vi "Set Port HW Entry.vi"(6 "InstrumentHandle_port":u32, 8 "boardresource":T1, 9 "portId":u32, 10 "boardId":u32, 11 "hw_data in":T2) -> (2 "duplicated":bool, 3 "hw_data out":T2)   [LabVIEW 2020, in "AIM664LV.lvlib"]
uses:
  AIM664LV.lvlib
  _controls/hwEntry_data.ctl
  _controls/hwEntryBoardHandleMap.ctl
  _controls/hwEntryBoardResource.ctl
  _controls/hwEntryPortResource.ctl
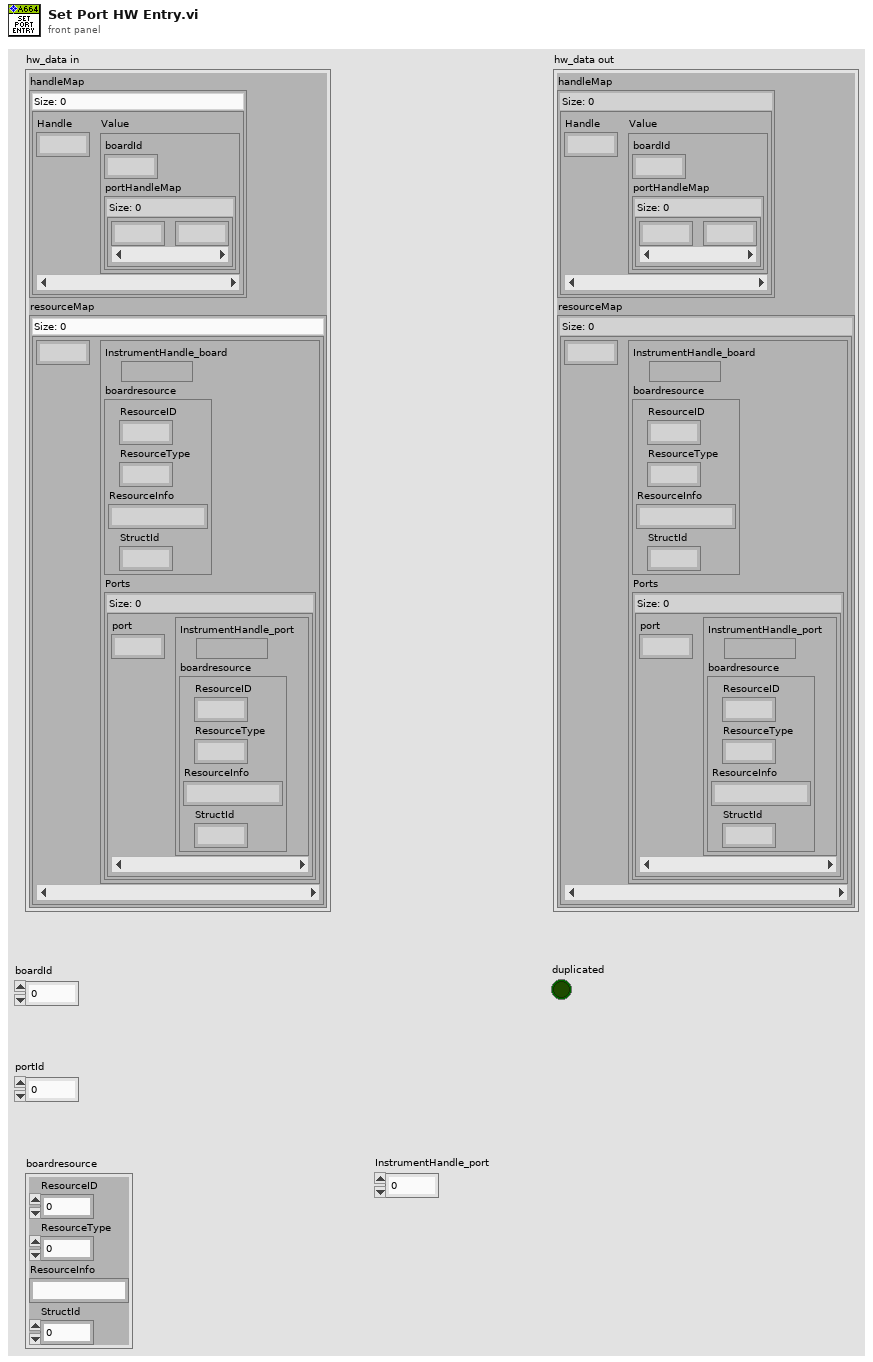
[diagram p1: front panel]
types:
  T1 = cluster{"ResourceID":u32, "ResourceType":u32, "ResourceInfo":string, "StructId":u32}
  T2 = typedef "AIM664LV.lvlib/hwEntry_data.ctl" = cluster{"handleMap":map{u32, T3}, "resourceMap":map{u32, T4}}
  T3 = typedef "AIM664LV.lvlib/hwEntryBoardHandleMap.ctl" = cluster{"boardId":u32, "portHandleMap":map{u32, u32}}
  T4 = typedef "AIM664LV.lvlib/hwEntryBoardResource.ctl" = cluster{"InstrumentHandle_board":u32, "boardresource":cluster{"ResourceID":u32, "ResourceType":u32, "ResourceInfo":string, "StructId":u32}, "Ports":map{u32, T5}}
  T5 = typedef "AIM664LV.lvlib/hwEntryPortResource.ctl" = cluster{"InstrumentHandle_port":u32, "boardresource":cluster{"ResourceID":u32, "ResourceType":u32, "ResourceInfo":string, "StructId":u32}}
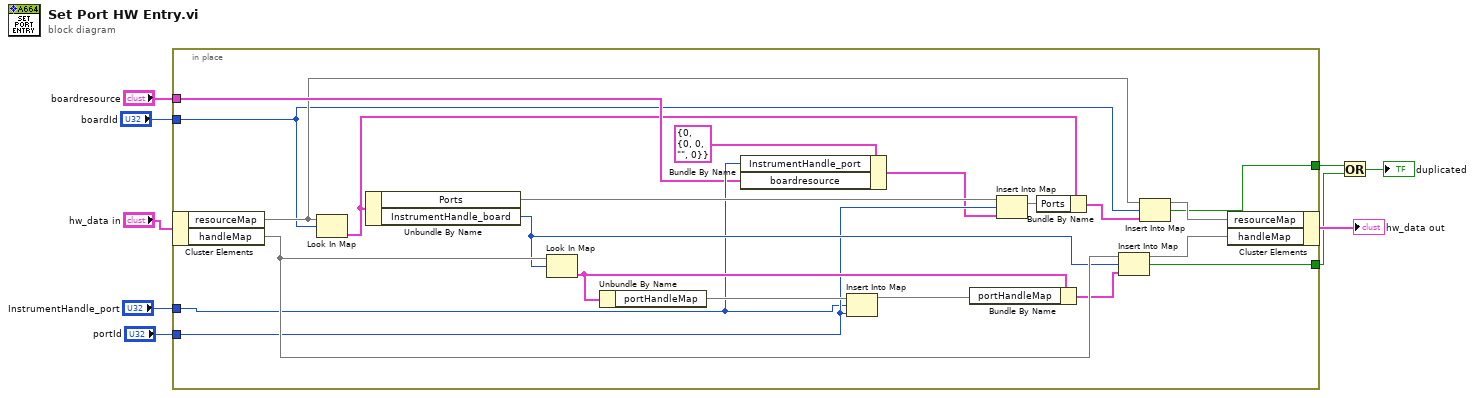
[diagram p0: block diagram]
diagram:
  n1 = in-place {
    in-place-border: "boardId" -> [w13]
    in-place-border: "InstrumentHandle_port" -> [w19]
    in-place-border: "boardresource" -> [w18]
    in-place-border: "portId" -> [w22]
    in-place-border: [w11] -> w2
    in-place-border: [w10] -> w1
    n2 = in-place-cluster #1("hw_data in") -> ("resourceMap"=w15:map{u32, T4}, "handleMap"=w29:map{u32, T3})
    n3 = Look In Map(map=w15, key=w13) -> (value=w17:T4)  [unwired: 1 in, 1 out]
    n4 = Unbundle By Name(w17) -> ("Ports"=w23:map{u32, T5}, "InstrumentHandle_board"=w28:u32)
    n5 = Look In Map(map=w29, key=w28) -> (value=w27:T3)  [unwired: 1 in, 1 out]
    n6 = Unbundle By Name(w27) -> ("portHandleMap"=w30:map{u32, u32})
    n7 = Bundle By Name(cluster=T5 {"InstrumentHandle_port"=0, "boardresource"={"ResourceID"=0, "ResourceType"=0, "ResourceInfo"="", "StructId"=0}} ("value"), "InstrumentHandle_port"=w19, "boardresource"=w18) -> (w20:T5)
    n8 = Insert Into Map(map in=w30, key=w19, value=w22) -> (map out=w26:map{u32, u32})  [unwired: 2 out]
    n9 = Bundle By Name(cluster=w27, "portHandleMap"=w26) -> (w25:T3)
    n10 = Insert Into Map(map in=w23, key=w22, value=w20) -> (map out=w16:map{u32, T5})  [unwired: 2 out]
    n11 = Bundle By Name(cluster=w17, "Ports"=w16) -> (w14:T4)
    n12 = Insert Into Map(map in=w29, key=w28, value=w25) -> (map out=w24:map{u32, T3}, key already included?=w10:bool)  [unwired: 1 out]
    n13 = Insert Into Map(map in=w15, key=w13, value=w14) -> (map out=w12:map{u32, T4}, key already included?=w11:bool)  [unwired: 1 out]
    n14 = in-place-cluster #1("resourceMap"=w12, "handleMap"=w24) -> (→"hw_data out":T2)
  }
  n15 = Or(x=w2, y=w1) -> (x .or. y?=→"duplicated":bool)
